vi "SaveWaveformData.vi"(6 "Registry":T16, 7 "data event data":T2, 8 "error in (no error)":errorcluster, 9 "dataflow type":T1, 10 "waveforms":waveform(sgl)[](array[waveform]), 11 "data event":T10) -> (0 "error out":errorcluster, 3 "data event data out":T2)   [LabVIEW 2017, in "CmsDataEventCreator.lvlib"]
uses:
  <vilib>/addons/InsightCM/Devices/Shared/Cms/CmsDataEventCreator/CmsDataEventCreator.lvlib
  <vilib>/addons/InsightCM/Devices/Shared/Cms/CmsDataEventCreator/controls/GroupRegistry.ctl
  <vilib>/addons/InsightCM/Devices/Shared/Cms/CmsDataEventCreator/controls/DataSetRegistry.ctl
  <vilib>/addons/InsightCM/Devices/Shared/Common/DataEvent/controls/DataSetType.ctl
  <vilib>/addons/InsightCM/Devices/Shared/Common/DataEventCreator/controls/Registry_Trend.ctl
  <vilib>/addons/InsightCM/Devices/Shared/Cms/CmsDataEventCreator/controls/DataEventConfig.ctl
  <vilib>/addons/InsightCM/Devices/Shared/Cms/CmsDataEventCreator/controls/AcqParams.ctl
  <vilib>/addons/InsightCM/Devices/Shared/Common/DataAccumulator/controls/AccumulationSettings.ctl
  <vilib>/addons/InsightCM/Devices/Shared/Common/DataAccumulator/controls/accumulationType.ctl
  <vilib>/addons/InsightCM/Devices/Shared/Common/DVRBuffer/controls/BufferLocation.ctl
  <vilib>/addons/PointValueMap/controls/PointMap.ctl
  <vilib>/addons/InsightCM/Devices/Shared/Common/DataEvent/controls/Event.ctl
  <vilib>/addons/InsightCM/MessageBus/Base/controls/DataEvent.ctl
  <vilib>/addons/InsightCM/MessageBus/Base/controls/KeyValuePair.ctl
  <vilib>/addons/InsightCM/Devices/Shared/Common/DataEvent/controls/DataSet.ctl
  <vilib>/addons/InsightCM/MessageBus/Base/controls/DataSetMetadata.ctl
  <vilib>/addons/InsightCM/MessageBus/Base/controls/TrendPoint.ctl
  <vilib>/addons/InsightCM/MessageBus/Base/controls/TrendAlarmUpdate.ctl
  <vilib>/addons/InsightCM/MessageBus/Base/controls/TrendAlarmTransition.ctl
  <vilib>/addons/InsightCM/Devices/Shared/Common/DataFlow/controls/Type.ctl
  <vilib>/addons/InsightCM/Devices/Shared/Common/DataFlow/DataFlow.lvlib
  <vilib>/addons/PointValueMap/PointValueMap.lvlib
  <vilib>/addons/InsightCM/Devices/Shared/Common/DataEvent/DataEvent.lvlib
  <vilib>/addons/InsightCM/Devices/Shared/Common/DataEventCreator/DataEventCreator.lvlib
  <vilib>/addons/InsightCM/Devices/Shared/Common/DataAccumulator/DataAccumulator.lvlib
  <vilib>/addons/InsightCM/Devices/Shared/Common/DVRBuffer/DVRBuffer.lvlib
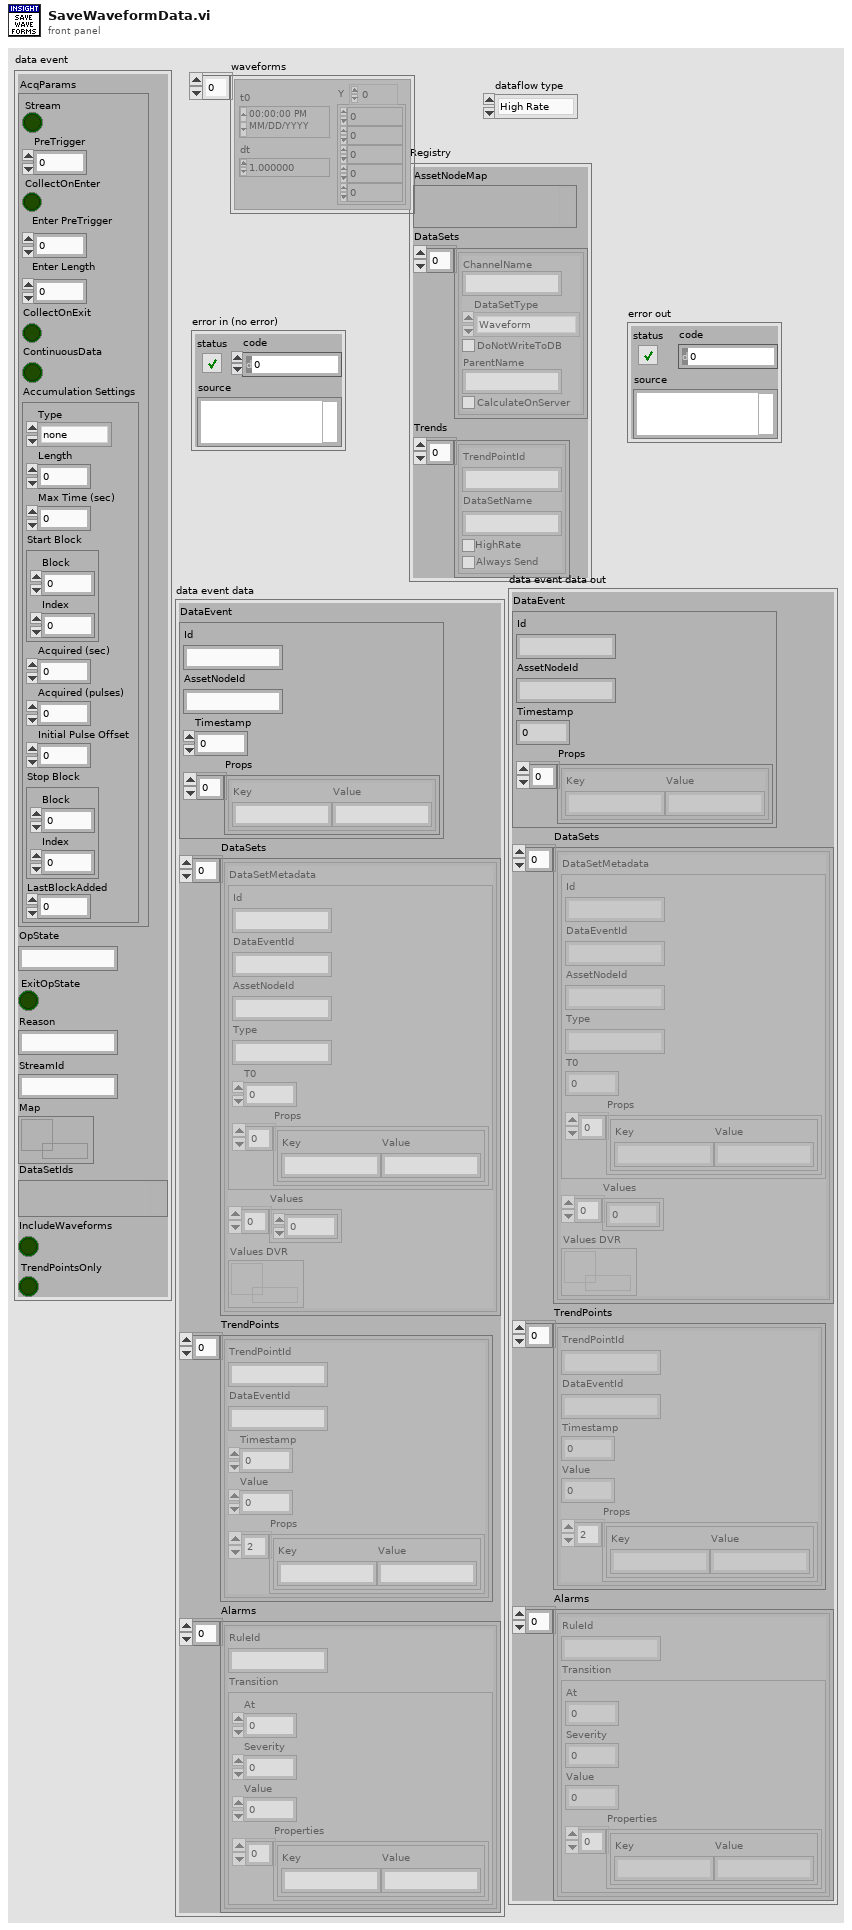
[diagram p1: front panel]
types:
  T1 = typedef "DataFlow.lvlib/Type.ctl" = enum16{"High Rate", "Low Rate", "Burst Mode"}
  T2 = typedef "DataEvent.lvlib/Event.ctl" = cluster{"DataEvent":T3, "DataSets":T5[], "TrendPoints":T7[], "Alarms":T8[]}
  T3 = typedef "DataEvent.ctl" = cluster{"Id":string, "AssetNodeId":string, "Timestamp":i64, "Props":T4[]}
  T4 = typedef "KeyValuePair.ctl" = cluster{"Key":string, "Value":string}
  T5 = typedef "DataEvent.lvlib/DataSet.ctl" = cluster{"DataSetMetadata":T6, "Values":sgl[], "Values DVR":refnum<data-value>}
  T6 = typedef "DataSetMetadata.ctl" = cluster{"Id":string, "DataEventId":string, "AssetNodeId":string, "Type":string, "T0":i64, "Props":T4[]}
  T7 = typedef "TrendPoint.ctl" = cluster{"TrendPointId":string, "DataEventId":string, "Timestamp":i64, "Value":dbl, "Props":T4[]}
  T8 = typedef "TrendAlarmUpdate.ctl" = cluster{"RuleId":string, "Transition":T9}
  T9 = typedef "TrendAlarmTransition.ctl" = cluster{"At":i64, "Severity":i32, "Value":dbl, "Properties":T4[]}
  T10 = typedef "CmsDataEventCreator.lvlib/DataEventConfig.ctl" = cluster{"AcqParams":T11, "OpState":string, "ExitOpState":bool, "Reason":string, "StreamId":string, "Map":T15, "DataSetIds":variant, "IncludeWaveforms":bool, "TrendPointsOnly":bool}
  T11 = typedef "CmsDataEventCreator.lvlib/AcqParams.ctl" = cluster{"Stream":bool, "PreTrigger":i32, "CollectOnEnter":bool, "Enter PreTrigger":i32, "Enter Length":dbl, "CollectOnExit":bool, "ContinuousData":bool, "Accumulation Settings":T12}
  T12 = typedef "DataAccumulator.lvlib/AccumulationSettings.ctl" = cluster{"Type":T13, "Length":dbl, "Max Time (sec)":dbl, "Start Block":T14, "Acquired (sec)":dbl, "Acquired (pulses)":i32, "Initial Pulse Offset":dbl, "Stop Block":T14, "LastBlockAdded":u32}
  T13 = typedef "DataAccumulator.lvlib/accumulationType.ctl" = enum16{"none", "seconds", "revolutions"}
  T14 = typedef "DVRBuffer.lvlib/BufferLocation.ctl" = cluster{"Block":u32, "Index":i32}
  T15 = typedef "PointValueMap.lvlib/PointMap.ctl" = refnum<data-value>
  T16 = typedef "CmsDataEventCreator.lvlib/GroupRegistry.ctl" = cluster{"AssetNodeMap":variant, "DataSets":T17[], "Trends":T19[]}
  T17 = typedef "CmsDataEventCreator.lvlib/DataSetRegistry.ctl" = cluster{"ChannelName":string, "DataSetType":T18, "DoNotWriteToDB":bool, "ParentName":string, "CalculateOnServer":bool}
  T18 = typedef "DataEvent.lvlib/DataSetType.ctl" = enum16{"Waveform", "SpeedProfile", "ThermalImage", "EmsaSweep"}
  T19 = typedef "DataEventCreator.lvlib/Registry_Trend.ctl" = cluster{"TrendPointId":string, "DataSetName":string, "HighRate":bool, "Always Send":bool}
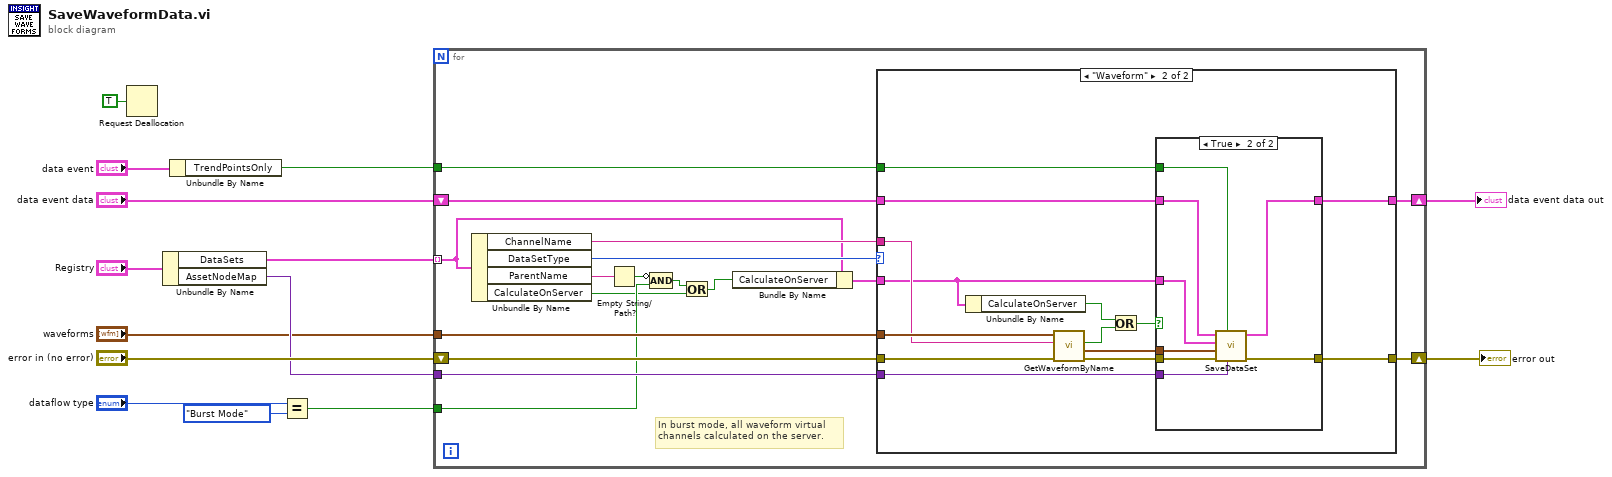
[diagram p0: block diagram]
diagram:
  n1 = Request Deallocation(TRUE ("flag")) -> ()
  n2 = Unbundle By Name("Registry") -> ("DataSets"=w12:T17[], "AssetNodeMap"=w10:variant)
  n3 = Unbundle By Name("data event") -> ("TrendPointsOnly"=w9:bool)
  n4 = Equal?(x="dataflow type", y=Type."Burst Mode") -> (x = y?=w1:bool)
  n5 = for {
    tunnel: "waveforms" -> [w30]
    tunnel: w12 -> [w22] mode=indexing
    shift-right: [w29] -> w11
    shift-left: "error in (no error)" -> [w31]
    tunnel: w10 -> [w25]
    shift-right: [w24] -> w6
    shift-left: "data event data" -> [w26]
    tunnel: w9 -> [w23]
    tunnel: w1 -> [w20]
    # "In burst mode, all waveform virtual\nchannels calculated on the server."
    n6 = Unbundle By Name(w22) -> ("ChannelName"=w28:string, "DataSetType"=w27:T18, "ParentName"=w18:string, "CalculateOnServer"=w16:bool)
    n7 = Empty String/Path?(string/path=w18) -> (empty?=w19:bool)
    n8 = Compound Arithmetic op=AND(invert w19, w20) -> (w17:bool)
    n9 = Or(x=w17, y=w16) -> (x .or. y?=w15:bool)
    n10 = Bundle By Name(cluster=w22, "CalculateOnServer"=w15) -> (w21:T17)
    n11 = case shown="\"Waveform\"" w27 {
      tunnel: w31 -> [w32 w38]
      tunnel: w30 -> [_ w47]
      tunnel: [w32 w46] -> w29
      tunnel: w28 -> [_ w45]
      tunnel: w26 -> [w33 w44]
      tunnel: w25 -> [_ w43]
      tunnel: w21 -> [_ w37]
      tunnel: [w33 w42] -> w24
      tunnel: w23 -> [_ w41]
      frame Default {
      }
      frame "Waveform" {
        n12 = Unbundle By Name(w37) -> ("CalculateOnServer"=w36:bool)
        n13 = call <vilib>:"GetWaveformByName.vi"("error in (no error)"=w38, "Channel Name"=w45, "Acq Waveforms"=w47) -> ("error out"=w40:errorcluster, "Waveform"=w39:waveform(sgl), "Found?"=w35:bool)  [unwired: 5 in, 1 out]
        n14 = Or(x=w36, y=w35) -> (x .or. y?=w34:bool)
        n15 = case shown="True" w34 {
          tunnel: w40 -> [w49 w57]
          tunnel: w39 -> [_ w56]
          tunnel: [w49 w51] -> w46
          tunnel: w44 -> [w48 w55]
          tunnel: w43 -> [_ w54]
          tunnel: w37 -> [_ w53]
          tunnel: [w48 w52] -> w42
          tunnel: w41 -> [_ w50]
          frame False {
          }
          frame True {
            n16 = call <vilib>:"SaveDataSet.vi"("AssetNodeMap"=w54, "do not write to database"=w50, "error in (no error)"=w57, "Waveform"=w56, "DataSetRegistry"=w53, "event in"=w55) -> ("error out"=w51:errorcluster, "event out"=w52:T2)  [unwired: 4 in]
          }
        }
      }
    }
  }
  "error out" <- w11
  "data event data out" <- w6
